vi "DRJHRTSRTJH.vi"   [LabVIEW 2016]
uses:
  <vilib>/rvi/eio/common/nirviEmuTemplateMethod_errors.vi
  <vilib>/eio/EIONode/EIONode.xnode
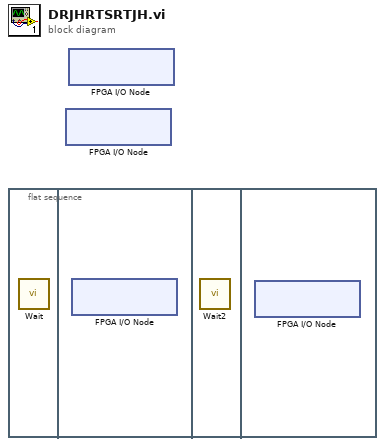
[diagram p0: block diagram]
diagram:
  n1 = flat-sequence {
    frame #0 {
      n2 = call "Wait"() -> ()  [unwired: 1 in, 1 out]
    }
    frame #1 {
      n3 = xnode "FPGA I/O Node"() -> ()  [unwired: 1 in, 2 out]
    }
    frame #2 {
      n4 = call "Wait2"() -> ()  [unwired: 1 in, 1 out]
    }
    frame #3 {
      n5 = xnode "FPGA I/O Node"() -> ()  [unwired: 1 in, 2 out]
    }
  }
  n6 = xnode "FPGA I/O Node"() -> ()  [unwired: 1 in, 2 out]
  n7 = xnode "FPGA I/O Node"() -> ()  [unwired: 1 in, 2 out]
